vi "FT10_Fornax Slider Status Command.vi"(9 "Slider Position":i32, 10 "Energy Channel ID":T1, 11 "Generator":T2="{\"Partition\":\"") -> (3 "JSON Command":string)   [LabVIEW 2015]
uses:
  Controls/Control_Fornax Generator.ctl
  Controls/Control_Fornax Energy Channel ID.ctl
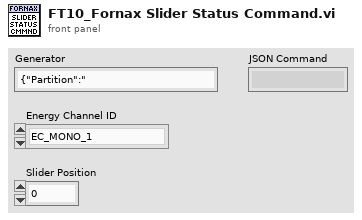
[diagram p1: front panel]
types:
  T1 = typedef "Control_Fornax Energy Channel ID.ctl" = enum16{"EC_MONO_1  ", "EC_BIPOLAR  ", "EC_MONO_2  ", "EC_ADVANCED  ", "EC_ADVANCED_ECUT  ", "EC_ADVANCED_DCUT  ", "EC_SHARED_COAG  ", "EC_INTERNAL_BIP_CAL  "}
  T2 = typedef "Control_Fornax Generator.ctl" = string
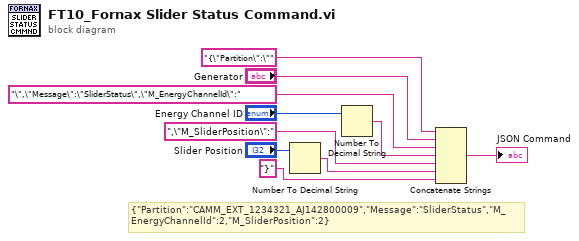
[diagram p0: block diagram]
diagram:
  # "{\"Partition\":\"CAMM_EXT_1234321_AJ142800009\",\"Message\":\"SliderStatus\",\"M_EnergyChannelId\":2,\"M_SliderPosition\":2}"
  n1 = Number To Decimal String(number="Slider Position") -> (decimal integer string=w9:string)  [unwired: 1 in]
  n2 = Number To Decimal String(number="Energy Channel ID") -> (decimal integer string=w7:string)  [unwired: 1 in]
  n3 = Concatenate Strings("{\"Partition\":\"", "Generator", "\",\"Message\":\"SliderStatus\",\"M_EnergyChannelId\":", w7, ",\"M_SliderPosition\":", w9, "}") -> (→"JSON Command":string)
